vi "Add Topology.vi"(6 "Append to Active?":bool, 7 "topology suffix (none)":string, 8 "error in (no error)":errorcluster, 9 "reset device (boolean value)":bool=TRUE, 10 "Topology":string, 11 "SLSC Switch in":refnum<class "SLSC Switch.lvclass">) -> (0 "error out":errorcluster, 3 "SLSC Switch out":refnum<class "SLSC Switch.lvclass">)   [LabVIEW 2015, in "SLSC Switch.lvlib" / "SLSC Switch.lvclass"]
uses:
  SLSC Switch.lvclass
  SLSC Switch.lvclass/SLSC Switch.ctl
  slscsl/slscsl.lvclass
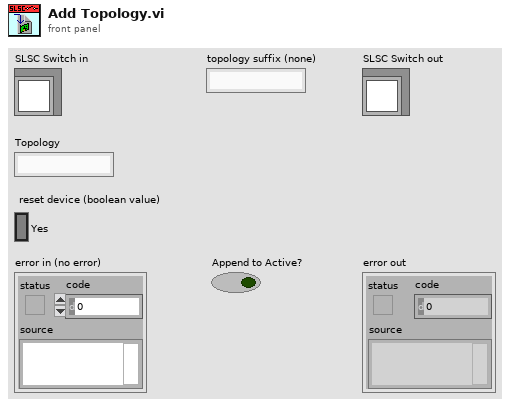
[diagram p1: front panel]
types:
  T1 = typedef "SLSC Switch.lvlib/SLSC Switch.lvclass/Topology.ctl" = cluster{"name":string, "InitialState":T2, "ChannelList":T3, "ConnectionList":T4[], "MuxList":cluster{"Src":string, "Dests":string[]}[]}
  T2 = typedef "SLSC Switch.lvlib/SLSC Switch.lvclass/JSON.InitialState.ctl" = cluster{"Open":string[], "Close":string[]}
  T3 = typedef "SLSC Switch.lvlib/SLSC Switch.lvclass/JSON.ChannelList.ctl" = cluster{"Names":string[]}
  T4 = typedef "SLSC Switch.lvlib/SLSC Switch.lvclass/JSON.ConnectionList.ctl" = cluster{"Src":string, "Dest":string, "Relays":string[]}
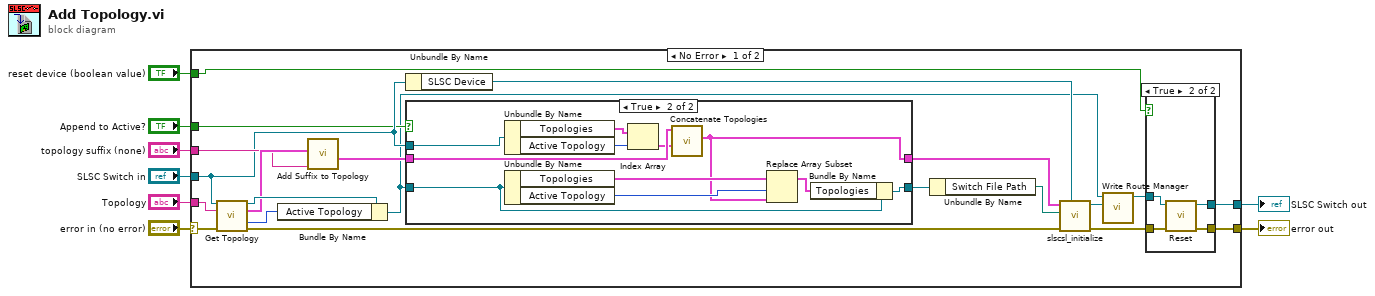
[diagram p0: block diagram]
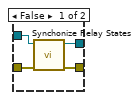
[diagram p3: hidden frame]
diagram:
  n1 = case shown="No Error" "error in (no error)" {
    selector: "error in (no error)" -> [w29 w52]
    tunnel: [w26 w52] -> w7
    tunnel: [w27 w51] -> w5
    tunnel: "SLSC Switch in" -> [w14 w51]
    tunnel: "reset device (boolean value)" -> [w23 _]
    tunnel: "Topology" -> [w28 _]
    tunnel: "topology suffix (none)" -> [w16 _]
    tunnel: "Append to Active?" -> [w12 _]
    frame No Error {
      n2 = call "Get Topology.vi"("SLSC Switch in"=w14, "Topology Name In"=w28, "error in (no error)"=w29) -> ("SLSC Switch out"=w20:refnum<class "SLSC Switch.lvclass">, "Topology out"=w17:T1, "Active Index"=w11:i32, "error out"=w18:errorcluster)  [unwired: 9 in]
      n3 = Bundle By Name(cluster=w20, "Active Topology"=w11) -> (w10:refnum<class "SLSC Switch.lvclass">)
      n4 = call "Add Suffix to Topology.vi"("topology suffix"=w16, "Topology in"=w17) -> ("Topology out"=w15:T1)  [unwired: 9 in]
      n5 = Unbundle By Name(w14) -> ("SLSC Device"=w19:refnum<k21>)
      n6 = case shown="True" w12 {
        tunnel: w15 -> [w31 w42]
        tunnel: w14 -> [_ w41]
        tunnel: [w31 w35] -> w13
        tunnel: w10 -> [w30 w34]
        tunnel: [w30 w32] -> w9
        frame False {
        }
        frame True {
          n7 = Unbundle By Name(w41) -> ("Topologies"=w38:T1[], "Active Topology"=w40:i32)
          n8 = Unbundle By Name(w34) -> ("Topologies"=w37:T1[], "Active Topology"=w36:i32)
          n9 = Index Array(array=w38, index=w40) -> (element=w39:T1)
          n10 = call "Concatenate Topologies.vi"("Topology B"=w39, "Topology A"=w42) -> ("Concatenated"=w35:T1)  [unwired: 9 in]
          n11 = Replace Array Subset(array=w37, new element=w35, index=w36) -> (w33:T1[])
          n12 = Bundle By Name(cluster=w34, "Topologies"=w33) -> (w32:refnum<class "SLSC Switch.lvclass">)
        }
      }
      n13 = Unbundle By Name(w9) -> ("Switch File Path"=w21:path)
      n14 = call "slscsl_initialize.vi"("deviceIdentifier"=w19, "error in (no error)"=w18, "shw file path"=w21, "Topology in"=w13) -> ("error out"=w25:errorcluster, "slscsl out"=w22:refnum<class "slscsl.lvclass">)  [unwired: 6 in]
      n15 = call "Write Route Manager.vi"("Route Manager.lvclass"=w22, "SLSC Switch in"=w10) -> ("SLSC Switch out"=w24:refnum<class "SLSC Switch.lvclass">)  [unwired: 9 in]
      n16 = case shown="True" w23 {
        tunnel: w25 -> [w46 w49]
        tunnel: [w45 w48] -> w26
        tunnel: [w44 w47] -> w27
        tunnel: w24 -> [w43 w50]
        frame False {
          n17 = call "Synchonize Relay States.vi"("error in (no error)"=w46, "SLSC Switch in"=w43) -> ("error out"=w45:errorcluster, "SLSC Switch out"=w44:refnum<class "SLSC Switch.lvclass">)  [unwired: 8 in]
        }
        frame True {
          n18 = call "Reset.vi"("error in (no error)"=w49, "SLSC Switch in"=w50) -> ("error out"=w48:errorcluster, "SLSC Switch out"=w47:refnum<class "SLSC Switch.lvclass">)  [unwired: 8 in]
        }
      }
    }
    frame Error {
    }
  }
  "error out" <- w7
  "SLSC Switch out" <- w5
